vi "12_500.vi"(11 "Numeric in":dbl) -> (3 "Numeric out":dbl)   [LabVIEW 2018]
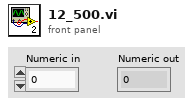
[diagram p1: front panel]
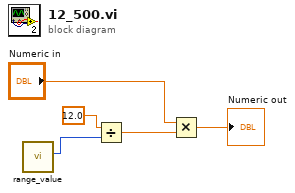
[diagram p0: block diagram]
diagram:
  n1 = call "range_value.vi"() -> ("NumBins"=w1:i32)  [unwired: 10 in, 1 out]
  n2 = Divide(x=12.0, y=w1) -> (x/y=w2:dbl)
  n3 = Multiply(x="Numeric in", y=w2) -> (x*y=→"Numeric out":dbl)
